vi "Hang Teleop.vi"(1 "Operator Buttons":bool[](array[boolean]), 2 "Driver Buttons":bool[](array[boolean]), 3 "Driver Axes":dbl[](array[numeric])) -> ()   [LabVIEW 2019]
uses:
  Implementation/Hang Operations.ctl
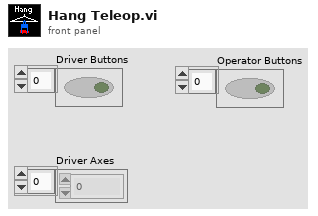
[diagram p1: front panel]
types:
  T1 = typedef "Hang Operations.ctl" = enum16{"Reserve", "Read Current", "Immediate", "Latch", "Un-Latch", "Color Wheel"}
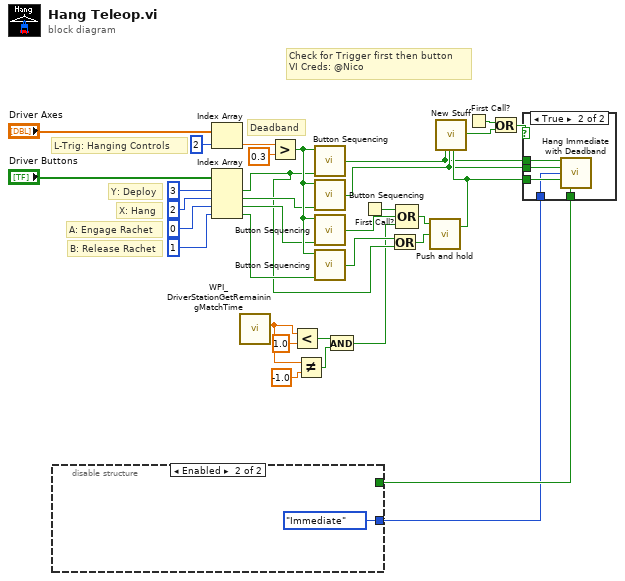
[diagram p0: block diagram]
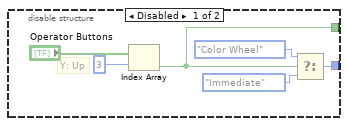
[diagram p2: hidden frame]
diagram:
  # "Check for Trigger first then button\nVI Creds: @Nico"
  # "Deadband"
  # "B: Release Rachet"
  # "A: Engage Rachet"
  # "L-Trig: Hanging Controls"
  # "X: Hang"
  # "Y: Deploy"
  n1 = disable-structure shown="Enabled" {
    disable-tunnel: [w35 Hang_Operations."Immediate" ("Operation")] -> w5
    disable-tunnel: [w34 _] -> w17
    frame Disabled {
      # "Y: Up"
      n2 = Index Array(array="Operator Buttons", index=3) -> (element=w34:bool)
      n3 = Select(t=Hang_Operations."Color Wheel" ("Operation"), s=w34, f=Hang_Operations."Immediate" ("Operation")) -> (s? t:f=w35:T1)
    }
    frame Enabled {
    }
  }
  n4 = Index Array(array="Driver Axes", index=2) -> (element=w26:dbl)
  n5 = Index Array(array="Driver Buttons", index #1=3 ("index"), index #2=2 ("index"), index #3=0 ("index"), index #4=1 ("index")) -> (element #1=w11:bool, element #2=w23:bool, element #3=w22:bool, element #4=w21:bool)
  n6 = call <vilib>:"WPI_DriverStationGetRemainingMatchTime.vi"() -> ("Match Time(s)"=w6:sgl)  [unwired: 10 in, 1 out]
  n7 = Greater?(x=w26, y=0.3) -> (0:w24:bool)
  n8 = Less?(x=w6, y=1.0) -> (x < y?=w9:bool)
  n9 = Not Equal?(x=w6, y=-1.0) -> (x != y?=w8:bool)
  n10 = call "Button Sequencing.vi"("2"=w11, "1"=w24) -> ("Boolean"=w18:bool)  [unwired: 4 in]
  n11 = call "Button Sequencing.vi"("2"=w23, "1"=w24) -> ("Boolean"=w19:bool)  [unwired: 4 in]
  n12 = call "Button Sequencing.vi"("2"=w22, "1"=w24) -> ("Boolean"=w3:bool)  [unwired: 4 in]
  n13 = call "Button Sequencing.vi"("2"=w21, "1"=w24) -> ("Boolean"=w13:bool)  [unwired: 4 in]
  n14 = And(x=w9, y=w8) -> (x .and. y?=w2:bool)
  n15 = First Call?() -> (First Call?: T/F=w4:bool)
  n16 = Or(x=w13, y=w11) -> (x .or. y?=w12:bool)
  n17 = Compound Arithmetic op=OR(w4, w3, w2) -> (w1:bool)
  n18 = call "Push and hold.vi"("Reset"=w12, "Input"=w1) -> ("Output"=w20:bool)  [unwired: 2 in]
  n19 = call "New Stuff.vi"("Variant 13"=w18, "Variant 6"=w19, "Variant 9"=w20) -> ("x != y?"=w16:bool)  [unwired: 24 in]
  n20 = First Call?() -> (First Call?: T/F=w15:bool)
  n21 = Or(x=w15, y=w16) -> (x .or. y?=w14:bool)
  n22 = case shown="True" w14 {
    tunnel: w20 -> [_ w45]
    tunnel: w19 -> [_ w44]
    tunnel: w18 -> [_ w43]
    tunnel: w5 -> [_ w42]
    tunnel: w17 -> [_ w41]
    frame False {
    }
    frame True {
      n23 = call "Hang Immediate with Deadband.vi"("Deploy?"=w43, "Hang?"=w44, "Operation"=w42, "Rachet Engaged?"=w45, "Deploy Color Wheel"=w41) -> ()  [unwired: 10 in, 1 out]
    }
  }
